vi "Yuval Algo.vi"() -> ()   [LabVIEW 2015]
uses:
  <resource>/objmgr/IMAQImage.rc
panel:
  out "Image Size":cluster{"x":i32, "y":i32}
  in  "stop":bool
  out "Time":u32
  out "Number of Matches (Shape Detection 1)":i32
  in  "Range (Threshold 1)":cluster{"Lower value":sgl, "Upper value":sgl}={"Lower value"=0.0, "Upper value"=195.0}
  out "Circles Calibrated (Shape Detection 1)":T1(array[cluster]) {"Position"."Y" format="%.2f"; "Position"."X" format="%.2f"}
  out "Circles (Shape Detection 1)":T1(array[cluster]) {"Position"."Y" format="%.2f"; "Position"."X" format="%.2f"}
  out "error out 2":errorcluster
  out "error out":errorcluster
  out "Image Out":T2(plugin-control)
  out "Image In":T2(plugin-control)
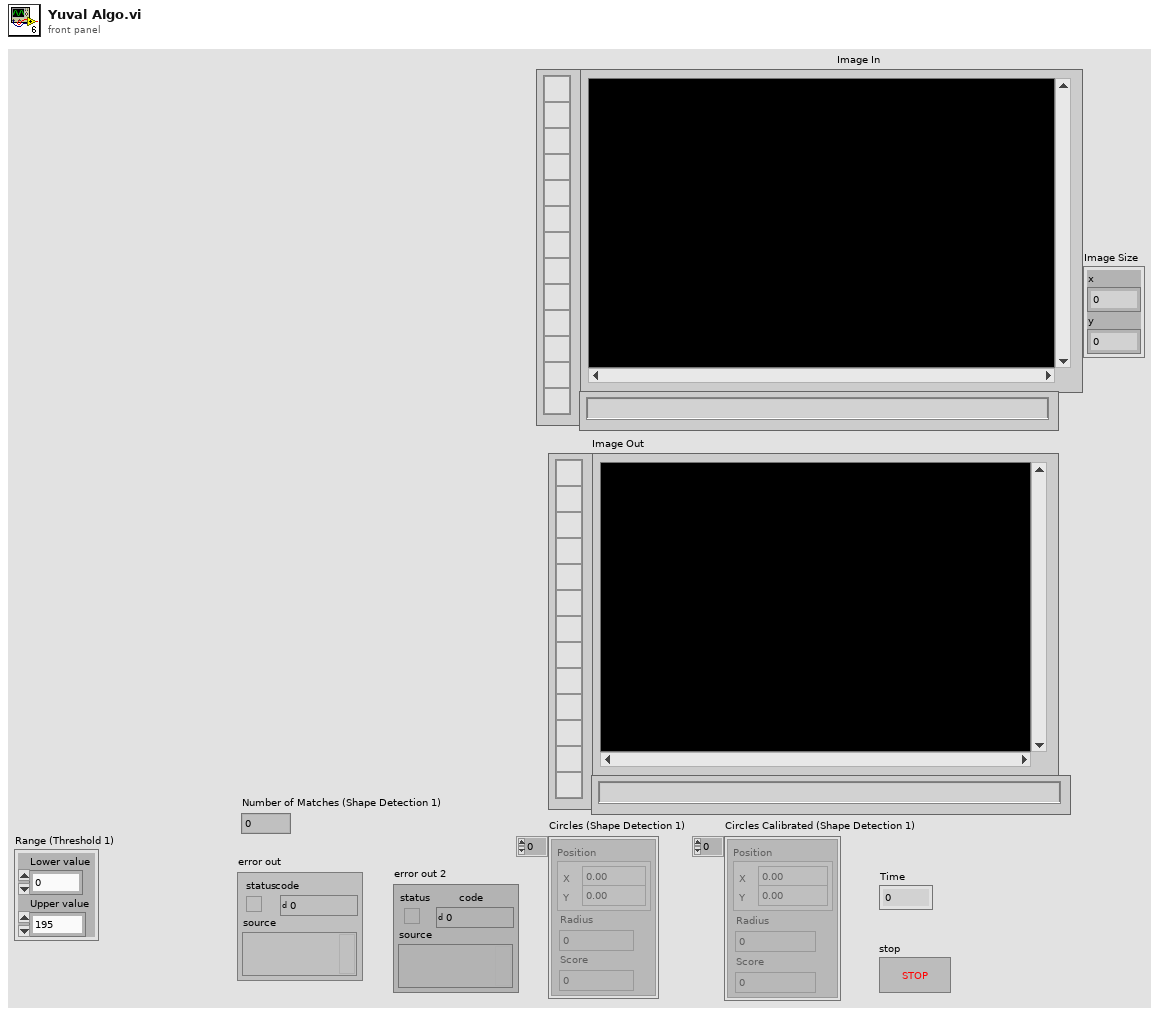
[diagram p1: front panel]
types:
  T1 = cluster{"Position":cluster{"X":sgl, "Y":sgl}, "Radius":dbl, "Score":dbl}[]
  T2 = typedef "IMAQ Image.ctl" = refnum<image>
  T3 = typedef "Image Type" = u32
  T4 = cluster{"Rotation":bool, "Scale":bool, "Occlusion":bool, "Range Settings":cluster{"Match Constraints":u32, "Min":dbl, "Max":dbl}[]}
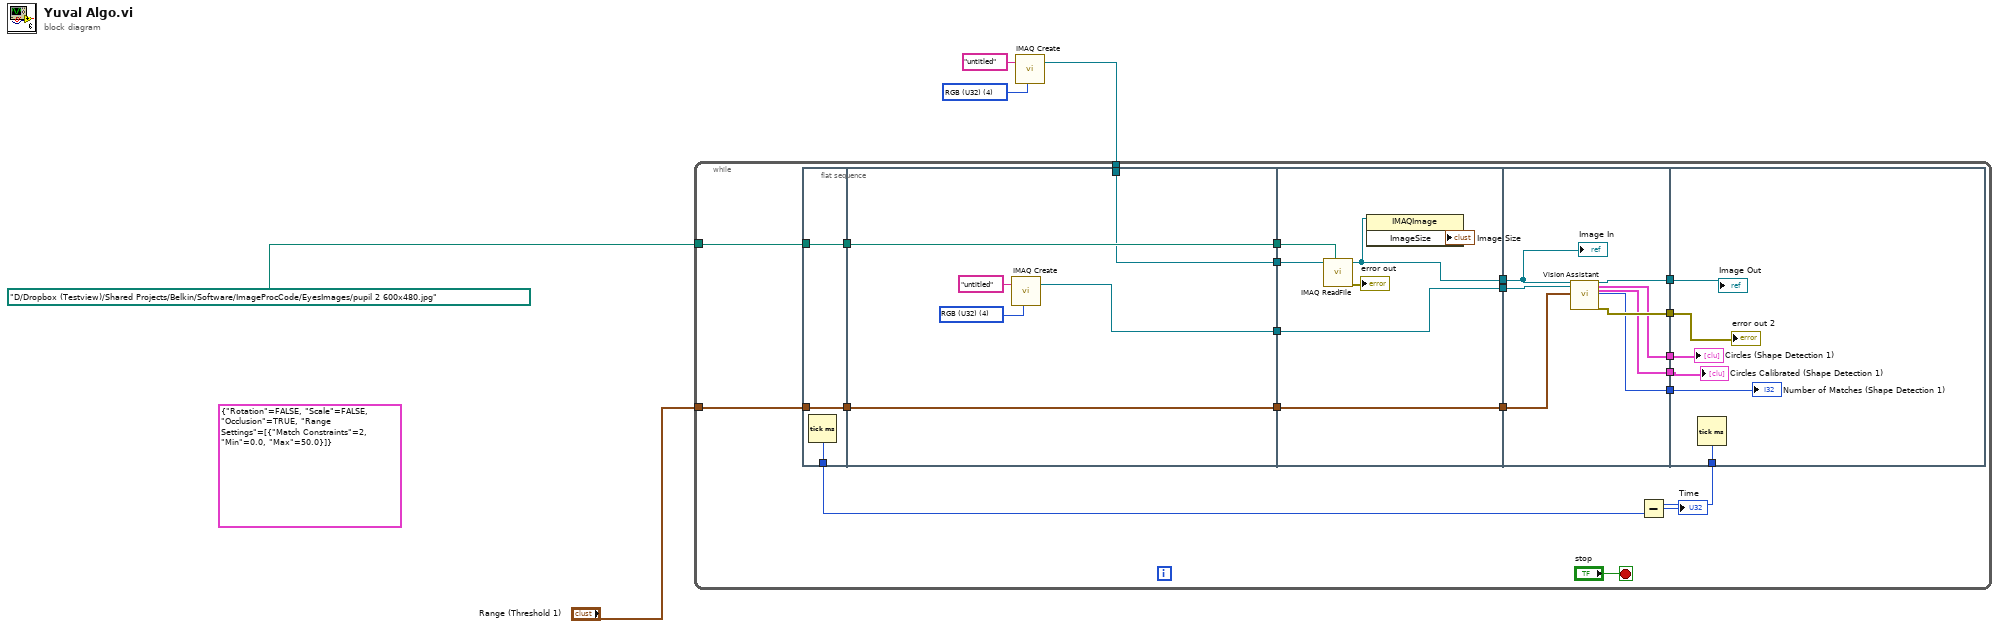
[diagram p0: block diagram]
diagram:
  w3 = T3 4 items=["Grayscale (U8)", "Grayscale (I16)", "Grayscale (SGL)", "Complex (CSG)", "RGB (U32)", "HSL (U32)", "RGB (U64)", "Grayscale (U16)"] ("Image Type")
  (unwired) T4 {"Rotation"=FALSE, "Scale"=FALSE, "Occlusion"=TRUE, "Range Settings"=[{"Match Constraints"=2, "Min"=0.0, "Max"=50.0}]} ("Match Options (Shape Detection 1)")
  n1 = call "IMAQ Create"("Image Name"="untitled", "Image Type"=w3) -> ("New Image"=w1:T2)  [unwired: 2 in, 2 out]
  n2 = while {
    tunnel: "Range (Threshold 1)" -> [w26]
    tunnel: path "D:/Dropbox (Testview)/Shared Projects/Belkin/Software/ImageProcCode/EyesImages/pupil 2 600x480.jpg" ("File Path") -> [w17]
    tunnel: w1 -> [w6]
    stop <- "stop" stop-if-true
    n3 = flat-sequence {
      tunnel: w17 -> [w28]
      tunnel: w26 -> [w29]
      tunnel: [w29] -> w11
      tunnel: [w28] -> w10
      tunnel: [w27] -> w9
      tunnel: [w35] -> w16
      tunnel: [w34] -> w15
      tunnel: [w33] -> w14
      tunnel: [w30] -> w13
      tunnel: w11 -> [w35]
      tunnel: w10 -> [w34]
      tunnel: w6 -> [w33]
      tunnel: [w42] -> w25
      tunnel: [w37] -> w19
      tunnel: w16 -> [w42]
      tunnel: w15 -> [w40]
      tunnel: w14 -> [w39]
      tunnel: w13 -> [w38]
      tunnel: [w38] -> w12
      tunnel: w25 -> [w49]
      tunnel: [w50] -> w24
      tunnel: [w45] -> w23
      tunnel: w19 -> [w43]
      tunnel: [w48] -> w18
      tunnel: w12 -> [w47]
      tunnel: [w46] -> w8
      tunnel: [w44] -> w7
      tunnel: w24 -> [w55]
      tunnel: w23 -> [w53]
      tunnel: [w56] -> w22
      tunnel: w18 -> [w51]
      tunnel: w8 -> [w54]
      tunnel: w7 -> [w52]
      frame #0 {
        n4 = Tick Count (ms)() -> (millisecond timer value=w27:u32)
      }
      frame #1 {
        w32 = T3 4 items=["Grayscale (U8)", "Grayscale (I16)", "Grayscale (SGL)", "Complex (CSG)", "RGB (U32)", "HSL (U32)", "RGB (U64)", "Grayscale (U16)"] ("Image Type")
        n5 = call "IMAQ Create"("Image Name"="untitled", "Image Type"=w32) -> ("New Image"=w30:T2)  [unwired: 2 in, 2 out]
      }
      frame #2 {
        n6 = call "IMAQ ReadFile"("File Path"=w40, "Image"=w39) -> ("error out"=→"error out":errorcluster, "Image Out"=w37:T2)  [unwired: 5 in, 3 out]
        n7 = property class="IMAQImage"(reference=w37) -> ("ImageSize"=→"Image Size":cluster{"x":i32, "y":i32})  [unwired: 1 in, 2 out]
      }
      frame #3 {
        n8 = call "Vision Assistant"("Image In"=w43, "Image Dst"=w47, "Range (Threshold 1)"=w49) -> ("Image Out"=w48:T2, "Circles (Shape Detection 1)"=w46:T1, "Circles Calibrated (Shape Detection 1)"=w45:T1, "Number of Matches (Shape Detection 1)"=w44:i32, "error out"=w50:errorcluster)  [unwired: 20 in]
        "Image In" <- w43
      }
      frame #4 {
        n9 = Tick Count (ms)() -> (millisecond timer value=w56:u32)
        "error out 2" <- w55
        "Circles (Shape Detection 1)" <- w54
        "Circles Calibrated (Shape Detection 1)" <- w53
        "Number of Matches (Shape Detection 1)" <- w52
        "Image Out" <- w51
      }
    }
    n10 = Subtract(x=w22, y=w9) -> (x-y=→"Time":u32)
  }
